vi "Acquisition Core.vi"(4 "Imaging Protocol":T1=enum."Live Imaging", 6 "Acquired z-plane index":i32, 8 "error in":errorcluster, 9 "AOL_Globals":T6={"Imaging Protocol"=enum."AOL Z-Stack", "Number of POI"=0, "Number of Miniscans"=0, "Number of Trials"=0, "Number of Cycles "=0, "# Averaged Frames"=0, "Laser power (%)"=0, "Pockels (V)"=0.0, "Acquisition Length (sec)"=0.0, "Fill time (us)"=0.0, "POI Dwell time (us)"=0.0, "Miniscan Dwell time per pixel (us)"=0.0, "PMT 1"=0.0, "PMT 2"=0.0, "Back Apperture (mA)"=200.0, "Frame Size"=0, "Center Frequency"=0.0, "Field of View (um)"=175.0, "Field of View (norm)"=0.0, "DwellTime (us)"=0.0, "Ref Dwell Time (us)"=0.0, "Wavelength (nm)"=0.0, "Zoom"=0.0, "AOL Z"=0.0, "AOL Mode"=enum."Raster", "GridXY"=0.0, "GridZ"=0.0, "TriggerPeriod (sec)"=0.0, "Number of Pixels in Miniscan"=0, "Experiment folder path"=path "", "X centre"=0.0, "Y centre"=0.0, "Angle (degrees)"=0.0, "Angle Xs (degrees)"=0.0, "Angle Ys (degrees)"=0.0, "Plane Mode"=0, "Threshold"=[], "Regenerate Chirps"=FALSE, "Rectangle ROI length (pixels)"=0, "Rectangle ROI height (pixels)"=0, "AOD fill"=4900, "StartupDelay"=0, "Samples Wait after Trigger"=5080, "Slip Cycle"=600000, "Add Cycle"=TRUE, "Functional Mode"=enum."Point", "Z Start"=0.0, "Z Stop"=0.0, "# Planes"=0, "Total Pixels"=0, "Variable Miniscan Pixels"=[], "Use Variable Length"=FALSE, "Use Variable Resolution"=FALSE, "Laser power (%) at Z Start"=0, "Laser power (%) at Z Stop"=0, "Ref Z Step"=0} {"Angle Ys (degrees)" format="%#.6g"; "Angle Xs (degrees)" format="%#.6g"; "Plane Mode" items=["XY Plane", "XZ Plane", "YZ Plane", "arbitraryplane"]; "Frame Size" items=["100X100"=100, "128X128"=128, "200X200"=200, "256X256"=256, "512X512"=512, "1024x1024"=1024, "2048x2048"=2048]; "Back Apperture (mA)" format="%#.6g"; "Pockels (V)" format="%#.6g"; "PMT 2" format="%#.6g"; "PMT 1" format="%#.6g"; "Angle (degrees)" format="%#.6g"; "POI Dwell time (us)" format="%#.6g"}, 10 "FPGA VI Ref":T2, 11 "Logging queue in":T10) -> (0 "error out":errorcluster, 1 "Logging queue element":T3={"Imaging Protocol"=enum."Live Imaging", "Number of Trials"=0, "Frame Size"=512, "# Averaged frames"=0, "Dwell time (us)"=0.0, "Index of Z-plane"=0, "Timelapse?"=FALSE, "Logging process is active"=FALSE, "Speed logging enabled"=FALSE, "tdms file ref"=refnum, "path"=path "", "Trial Number"=0, "Expected # points acquired"=FALSE, "Manually stopped"=FALSE, "Last trial"=FALSE, "Ch0 data"=[], "Ch1 data"=[], "Ref Data"=[], "Ref Frame Time"=[], "Image Time"=[], "Continuous Time"=[], "Ref X Length"=0, "Ref Y Length"=0, "# Ref Averaged frames"=0, "Ref Dwell time (us)"=0.0, "Points acquired"={"Ch0 last trial"=0, "Ch1 last trial"=0, "All trials"=0}, "HW Timings File"=refnum} {"Ref Dwell time (us)" format="%#.6g"; "Frame Size" items=["100X100"=100, "128X128"=128, "200X200"=200, "256X256"=256, "512X512"=512, "1024x1024"=1024, "2048x2048"=2048]; "Dwell time (us)" format="%#.6g"})   [LabVIEW 2020]
uses:
  Typedefs/Data queue ref.ctl
  Typedefs/Logging queue element.ctl
  Typedefs/Imaging Protocols enum.ctl
  Typedefs/Frame Size.ctl
  Typedefs/Acquired points count.ctl
  Typedefs/Controls/AOL_Globals.ctl
  Typedefs/AOL modes.ctl
  Typedefs/Plane Mode.ctl
  Typedefs/Functional Mode.ctl
  RIG-SPECIFIC FILES/FPGA Refs/FPGA Ref.ctl
  Typedefs/Read Write Enum.ctl
  Video Rec Signaling/typedefs/Functions enum.ctl
  Global Variables/General Globals.vi
panel:
  out "subVI exec time":u32
  out "VI exec time":u32
  out "Elements Remaining in FIFO":u32
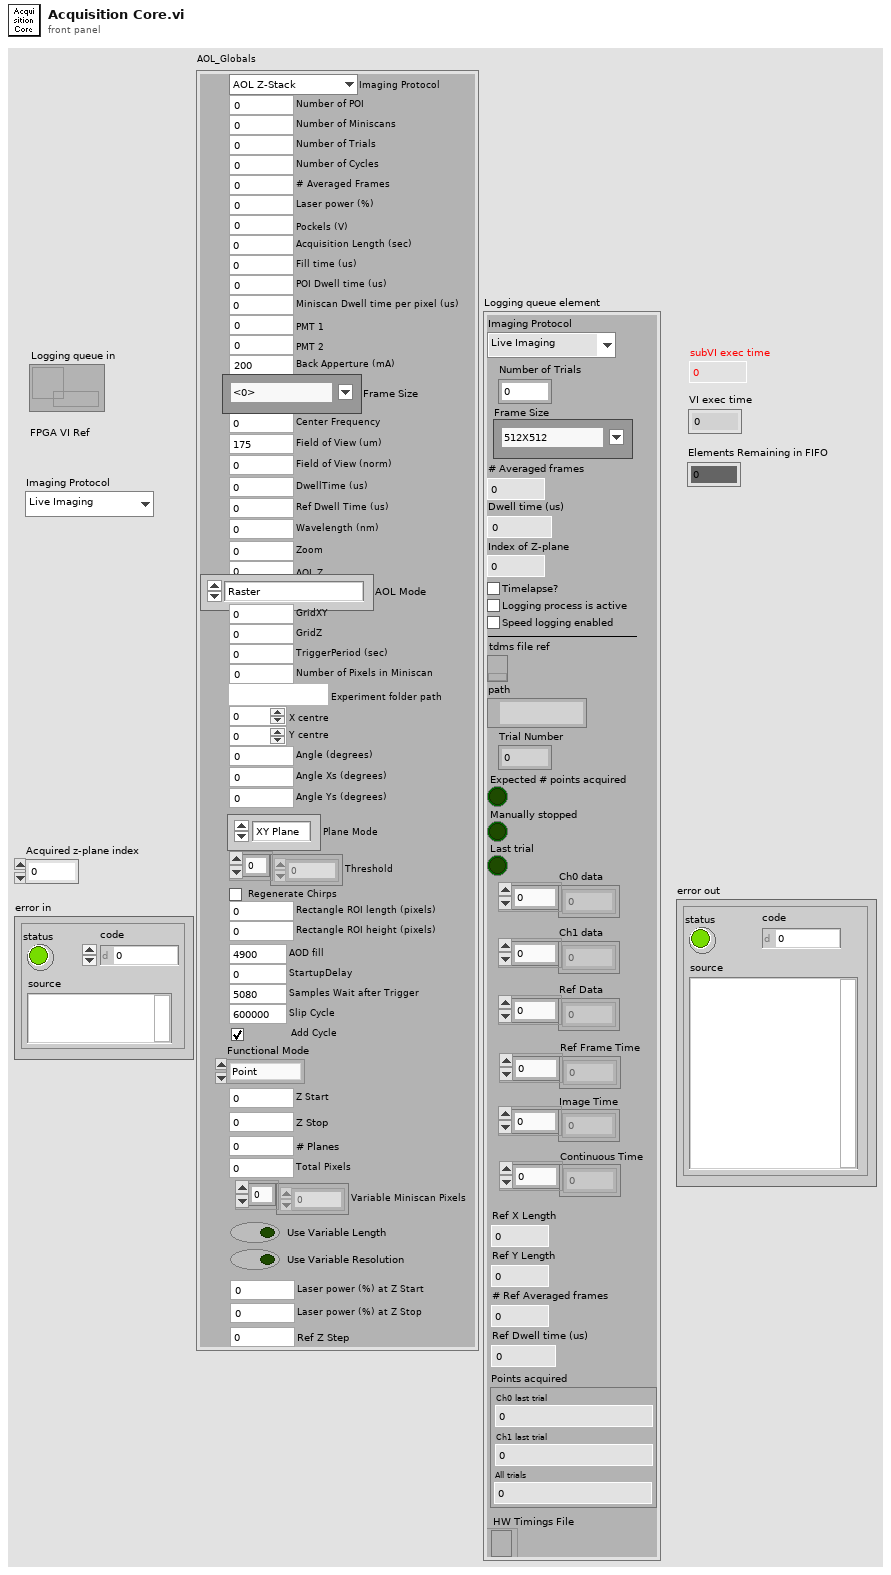
[diagram p1: front panel]
types:
  T1 = typedef "Imaging Protocols enum.ctl" = enum16{"AOL Z-Stack", "Motor Z Stack", "Parameter Sweep", "Functional Acquisition", "Single Plane Acquisition", "Volume Acquisition", "Live Imaging", "Live Plane Imaging", "Live Volume Imaging"}
  T2 = typedef "FPGA Ref.ctl" = refnum<k20>
  T3 = typedef "Logging queue element.ctl" = cluster{"Imaging Protocol":T1, "Number of Trials":u16, "Frame Size":T4, "# Averaged frames":u16, "Dwell time (us)":dbl, "Index of Z-plane":i32, "Timelapse?":bool, "Logging process is active":bool, "Speed logging enabled":bool, "tdms file ref":refnum<k34>, "path":path, "Trial Number":i32, "Expected # points acquired":bool, "Manually stopped":bool, "Last trial":bool, "Ch0 data":u32[], "Ch1 data":u32[], "Ref Data":u32[], "Ref Frame Time":u64[], "Image Time":u64[], "Continuous Time":u64[], "Ref X Length":u16, "Ref Y Length":u16, "# Ref Averaged frames":u16, "Ref Dwell time (us)":dbl, "Points acquired":T5, "HW Timings File":refnum<file>}
  T4 = typedef "Frame Size.ctl" = u16
  T5 = typedef "Acquired points count.ctl" = cluster{"Ch0 last trial":u64, "Ch1 last trial":u64, "All trials":u64}
  T6 = typedef "AOL_Globals.ctl" = cluster{"Imaging Protocol":T1, "Number of POI":u16, "Number of Miniscans":u16, "Number of Trials":u16, "Number of Cycles ":u64, "# Averaged Frames":u16, "Laser power (%)":u8, "Pockels (V)":dbl, "Acquisition Length (sec)":dbl, "Fill time (us)":dbl, "POI Dwell time (us)":dbl, "Miniscan Dwell time per pixel (us)":dbl, "PMT 1":dbl, "PMT 2":dbl, "Back Apperture (mA)":dbl, "Frame Size":T4, "Center Frequency":dbl, "Field of View (um)":dbl, "Field of View (norm)":dbl, "DwellTime (us)":dbl, "Ref Dwell Time (us)":dbl, "Wavelength (nm)":dbl, "Zoom":dbl, "AOL Z":dbl, "AOL Mode":T7, "GridXY":dbl, "GridZ":dbl, "TriggerPeriod (sec)":dbl, "Number of Pixels in Miniscan":u16, "Experiment folder path":path, "X centre":dbl, "Y centre":dbl, "Angle (degrees)":dbl, "Angle Xs (degrees)":dbl, "Angle Ys (degrees)":dbl, "Plane Mode":T8, "Threshold":u16[], "Regenerate Chirps":bool, "Rectangle ROI length (pixels)":u16, "Rectangle ROI height (pixels)":u16, "AOD fill":u16, "StartupDelay":i32, "Samples Wait after Trigger":u16, "Slip Cycle":u32, "Add Cycle":bool, "Functional Mode":T9, "Z Start":dbl, "Z Stop":dbl, "# Planes":i32, "Total Pixels":i32, "Variable Miniscan Pixels":u16[], "Use Variable Length":bool, "Use Variable Resolution":bool, "Laser power (%) at Z Start":u8, "Laser power (%) at Z Stop":u8, "Ref Z Step":i8}
  T7 = typedef "AOL modes.ctl" = enum16{"Raster", "Structural", "Pointing", "Mini Scan", "Alignment"}
  T8 = typedef "Plane Mode.ctl" = u16
  T9 = typedef "Functional Mode.ctl" = enum16{"Point", "Line", "Patch", "Plane", "Volume"}
  T10 = typedef "Data queue ref.ctl" = refnum<queue>
  T11 = enum16{"Obtain queue", "Call window", "Call & send signal", "Release queue"}
  T12 = typedef "Read Write Enum.ctl" = enum16{"Read", "Write"}
  T13 = typedef "Functions enum.ctl" = enum16{"Create", "Start", "Write", "Stop", "Clear"}
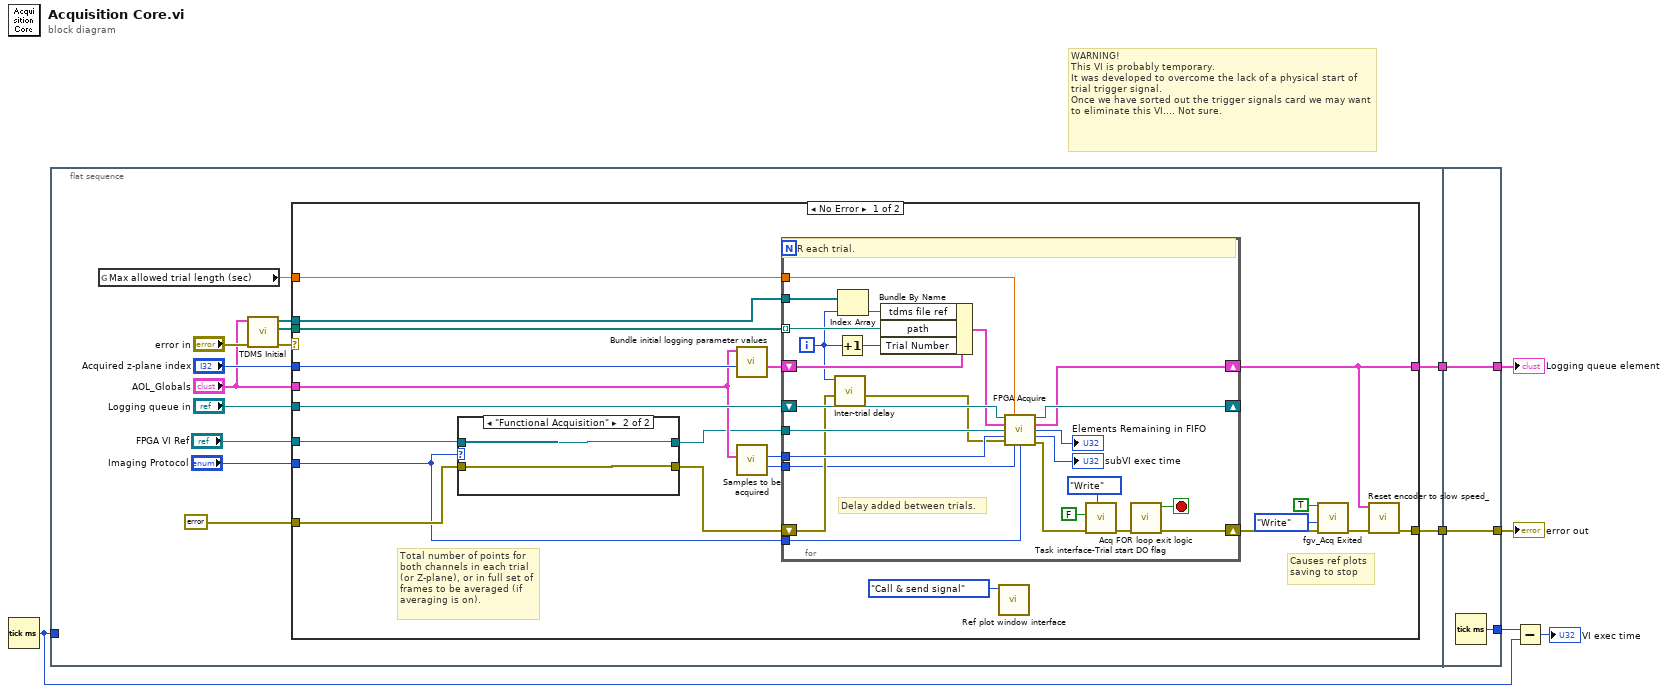
[diagram p0: block diagram]
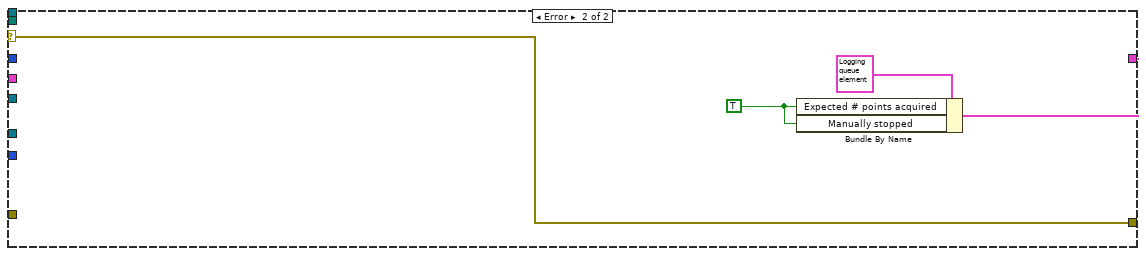
[diagram p3: hidden frame]
diagram:
  # "WARNING!\nThis VI is probably temporary.\nIt was developed to overcome the lack of a physical start of trial trigger signal.\nOnce we have sorted out the trigger signals card we may want to eliminate this VI.... Not sure."
  n1 = Tick Count (ms)() -> (millisecond timer value=w1:u32)
  n2 = flat-sequence {
    tunnel: w1 -> [_]
    tunnel: [w16] -> w5
    tunnel: [w11] -> w2
    tunnel: [w77] -> w7
    tunnel: [w76] -> w4
    tunnel: w5 -> [w76]
    tunnel: [w75] -> w3
    tunnel: w2 -> [w75]
    frame #0 {
      n3 = global read "General Globals.vi" "Max allowed trial length (sec)"() -> (w12:dbl)
      n4 = call "TDMS Initial.vi"("error in"="error in", "AOL_Globals"="AOL_Globals") -> ("error IO"=w19:errorcluster, "TDMS file paths OR experiment folder path"=w17:path[], "Functional imaging TDMS file references"=w18:refnum<k34>[])  [unwired: 7 in]
      n5 = case shown="No Error" w19 {
        selector: w19 -> [_ w71]
        tunnel: "Logging queue in" -> [w41 _]
        tunnel: w18 -> [w40 _]
        tunnel: w17 -> [w39 _]
        tunnel: [w33 w71] -> w11
        tunnel: "AOL_Globals" -> [w27 _]
        tunnel: "Acquired z-plane index" -> [w36 _]
        tunnel: [w32 w72] -> w16
        tunnel: w12 -> [w34 _]
        tunnel: "FPGA VI Ref" -> [w23 _]
        tunnel: "Imaging Protocol" -> [w21 _]
        tunnel: errorcluster {"status"=FALSE, "code"=0, "source"=""} ("error out") -> [w22 _]
        frame No Error {
          # "Total number of points for both channels in each trial (or Z-plane), or in full set of frames to be averaged (if averaging is on)."
          # "Causes ref plots\nsaving to stop"
          n6 = case shown="\"Functional Acquisition\"" w21 {
            tunnel: [w43 w45] -> w25
            tunnel: [w42 w44] -> w24
            tunnel: w23 -> [w43 w45]
            tunnel: w22 -> [w42 w44]
            frame Default {
            }
            frame "Functional Acquisition" {
            }
          }
          n7 = call "Bundle initial logging parameter values.vi"("Index of Z plane"=w36, "AOL_Globals IN"=w27) -> ("Logging queue element"=w38:T3)  [unwired: 9 in]
          n8 = call "Samples to be acquired.vi"("AOL_Globals"=w27) -> ("Number of Ref samples to be acquired"=w35:u32, "Number of samples to be acquired (points in frame x Ch. x Av.)"=w37:u64)  [unwired: 8 in, 1 out]
          n9 = for {
            shift-right: [w61] -> _
            shift-left: w41 -> [w66]
            tunnel: w37 -> [w65]
            tunnel: w40 -> [w69]
            tunnel: w39 -> [w64] mode=indexing
            shift-right: [w50] -> w30
            shift-left: w24 -> [w48]
            tunnel: w25 -> [w62]
            tunnel: w35 -> [w47]
            tunnel: w34 -> [w57]
            shift-right: [w53] -> w32
            shift-left: w38 -> [w63]
            tunnel: w21 -> [w46]
            i -> [w56]
            stop <- w67 stop-if-true
            # "Delay added between trials."
            # "FOR each trial."
            n10 = call "Inter-trial delay.vi"("error in"=w48, "Trial index"=w56) -> ("error out"=w49:errorcluster)  [unwired: 9 in]
            n11 = Increment(x=w56) -> (x+1=w70:i32)
            n12 = Index Array(array=w69, index=w56) -> (element=w68:refnum<k34>)
            n13 = Bundle By Name(cluster=w63, "tdms file ref"=w68, "path"=w64, "Trial Number"=w70) -> (w60:T3)
            n14 = call "FPGA Acquire.vi"("Logging queue in"=w66, "Max allowed trial length (sec)"=w57, "Logging queue element IN"=w60, "FPGA Ref"=w62, "Target number of points"=w65, "error in (no error)"=w49, "Total number of Ref points"=w47, "Imaging Protocol"=w46) -> ("Logging queue out"=w61:T10, "Logging queue element OUT"=w53:T3, "Elements Remaining"=→"Elements Remaining in FIFO":u32, "VI exec time"=→"subVI exec time":u32, "error out"=w52:errorcluster)  [unwired: 3 in]
            n15 = call "Task interface-Trial start DO flag.vi"("Function"=Functions_enum."Write", "error in"=w52, "DO value"=FALSE) -> ("error out"=w51:errorcluster)  [unwired: 8 in]
            n16 = call "Acq FOR loop exit logic.vi"("error in (no error)"=w51) -> ("error out (dupl)"=w50:errorcluster, "Stop acquisition FOR loop"=w67:bool)  [unwired: 9 in]
          }
          n17 = call "Ref plot window interface.vi"("Function"=T11."Call & send signal") -> ()  [unwired: 9 in, 2 out]
          n18 = call "fgv_Acq Exited.vi"("error in (no error)"=w30, "Function"=Read_Write_Enum."Write", "Acquisition completed"=TRUE ("Timelapse?")) -> ("error out"=w29:errorcluster)  [unwired: 7 in, 1 out]
          n19 = call "Reset encoder to slow speed_.vi"("error in (no error)"=w29, "Logging queue element"=w32) -> ("error out"=w33:errorcluster)  [unwired: 9 in]
        }
        frame Error {
          w74 = TRUE ("Manually stopped")
          n20 = Bundle By Name(cluster=T3 {"Imaging Protocol"=enum."AOL Z-Stack", "Number of Trials"=0, "Frame Size"=0, "# Averaged frames"=0, "Dwell time (us)"=0.0, "Index of Z-plane"=0, "Timelapse?"=FALSE, "Logging process is active"=FALSE, "Speed logging enabled"=FALSE, "tdms file ref"=refnum, "path"=path "", "Trial Number"=0, "Expected # points acquired"=FALSE, "Manually stopped"=FALSE, "Last trial"=FALSE, "Ch0 data"=[], "Ch1 data"=[], "Ref Data"=[], "Ref Frame Time"=[], "Image Time"=[], "Continuous Time"=[], "Ref X Length"=0, "Ref Y Length"=0, "# Ref Averaged frames"=0, "Ref Dwell time (us)"=0.0, "Points acquired"={"Ch0 last trial"=0, "Ch1 last trial"=0, "All trials"=0}, "HW Timings File"=refnum} ("Logging queue element"), "Expected # points acquired"=w74, "Manually stopped"=w74) -> (w72:T3)
        }
      }
    }
    frame #1 {
      n21 = Tick Count (ms)() -> (millisecond timer value=w77:u32)
    }
  }
  n22 = Subtract(x=w7, y=w1) -> (x-y=→"VI exec time":u32)
  "Logging queue element" <- w4
  "error out" <- w3
